vi "20TILMMonitor.vi"   [LabVIEW 2016]
uses:
  Instrument_Setup.vi
  Global/Global Variables/Data_Display_global.vi
  Equipment/Mercury iXX/Public/Libraries/Level Meter/Open/Open Level Meter Device.vi
  Equipment/Mercury iXX/Public/Libraries/Level Meter/Signals/Read/Probe Level Helium (Read).vi
  Equipment/Mercury iXX/Public/Libraries/Temperature/Open/Open Temperature Device.vi
  Equipment/Mercury iXX/Public/Libraries/Temperature/Signals/Read/Temperature (Read).vi
  Equipment/Mercury iXX/Public/Libraries/Auxiliary/Open/Open Auxiliary Device.vi
  Equipment/Mercury iXX/Public/Libraries/Auxiliary/Signals/Read/Percent Open (Read).vi
  Equipment/Mercury iXX/Public/Libraries/Pressure/Open/Open Pressure Device.vi
  Equipment/Mercury iXX/Public/Libraries/Pressure/Signals/Read/Pressure (Read).vi
  Equipment/Mercury iXX/Mercury iXX.lvlib
  Equipment/Mercury iXX/Public/Libraries/Pressure.lvlib
  Equipment/Mercury iXX/Public/Libraries/Auxiliary.lvlib
  Equipment/Mercury iXX/Public/Libraries/Temperature.lvlib
  Equipment/Mercury iXX/Public/Libraries/Level Meter.lvlib
types:
  T1 = typedef "Mercury iXX.lvlib/Mercury Reference.ctl" = cluster{"Comms":refnum<visa-resource-name>, "Device ID":string[], "Comms Layer":T2, "Command":string, "Query reference":T3}
  T2 = typedef "Mercury iXX.lvlib/Comms Transport Layer.ctl" = enum16{"Ethernet TCP/IP", "USB", "ISOBus - RS-232", "GPIB"}
  T3 = typedef "Mercury iXX.lvlib/Query Dynamic Reference.ctl" = refnum<vi>
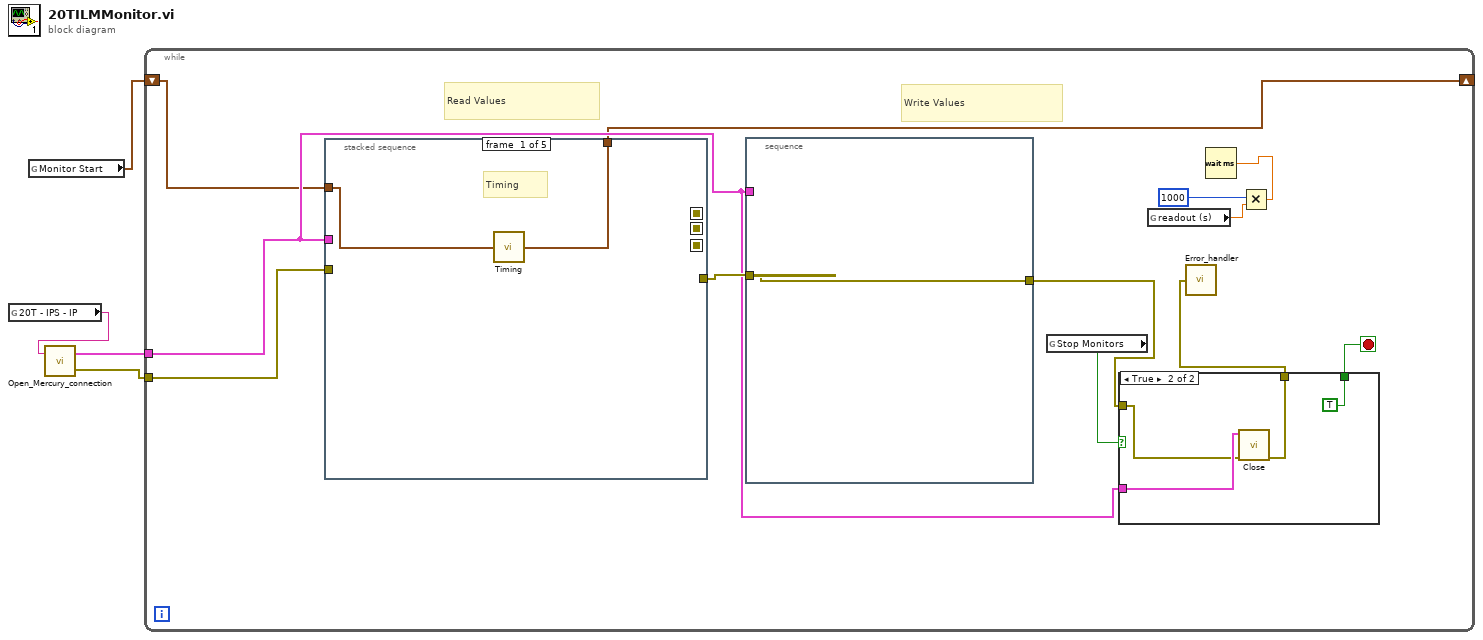
[diagram p0: block diagram]
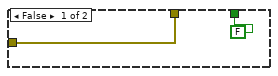
[diagram p2: hidden frame]
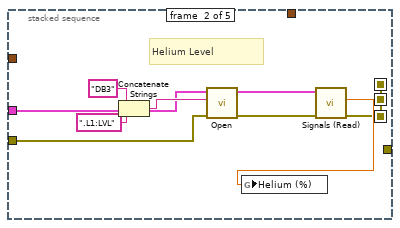
[diagram p3: hidden frame]
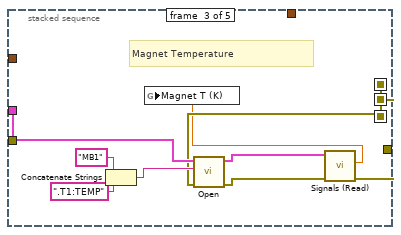
[diagram p4: hidden frame]
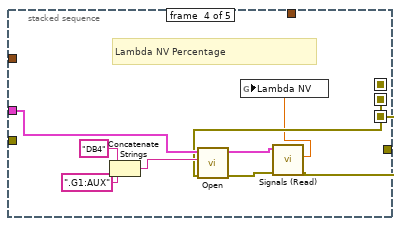
[diagram p5: hidden frame]
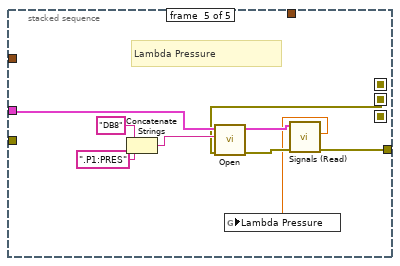
[diagram p6: hidden frame]
diagram:
  n1 = global read "Instrument_Setup.vi" "20T - IPS - IP"() -> (w2:string)
  n2 = global read "Data_Display_global.vi" "Monitor Start"() -> (w1:timestamp)
  n3 = call "Open_Mercury_connection.vi"("IP Address"=w2) -> ("error out"=w3:errorcluster, "Mercury Reference Out"=w4:T1)  [unwired: 1 in]
  n4 = while {
    tunnel: w4 -> [w7]
    tunnel: w3 -> [w16]
    shift-right: [w5] -> _
    shift-left: w1 -> [w6]
    stop <- w11 stop-if-true
    # "Write Values"
    # "Read Values"
    n5 = stacked-sequence {
      seq-local: [_ w26 _ _ _] -> [_ _ w37 _ _]
      seq-local: [_ _ w36 _ _] -> [_ _ _ w48 w57]
      seq-local: [_ _ _ w45 _] -> [_ _ _ _ _]
      tunnel: w7 -> [_ w29 w38 w49 w58]
      tunnel: w16 -> [_ w28 _ _ _]
      tunnel: [_ _ _ _ w53] -> w15
      tunnel: w6 -> [w25 _ _ _ _]
      tunnel: [w24 _ _ _ _] -> w5
      frame #0 {
        # "Timing"
        n6 = call "Timing.vi"("start time (s)"=w25) -> ("last reading (s)"=w24:timestamp)
      }
      frame #1 {
        # "Helium Level"
        n7 = Concatenate Strings("DB3", ".L1:LVL" ("Device Identifier")) -> (w32:string)
        n8 = call-poly "Open.vi"("error in (no error)"=w28, "Device Identifier"=w32, "Mercury Reference In"=w29) -> ("error out"=w34:errorcluster, "Mercury Reference Out"=w33:T1)  [unwired: 1 in, 6 out]
        n9 = call-poly "Signals (Read).vi"("error in"=w34, "Mercury Reference In"=w33) -> ("error out"=w26:errorcluster, "Level"=w27:dbl)  [unwired: 5 in, 3 out]
        n10 = global write "Data_Display_global.vi" "Helium (%)"(w27) -> ()
      }
      frame #2 {
        # "Magnet Temperature"
        n11 = Concatenate Strings("MB1", ".T1:TEMP" ("Device Identifier")) -> (w41:string)
        n12 = call-poly "Open.vi"("error in (no error)"=w37, "Device Identifier"=w41, "Mercury Reference In"=w38) -> ("error out"=w43:errorcluster, "Mercury Reference Out"=w42:T1)  [unwired: 1 in, 6 out]
        n13 = call-poly "Signals (Read).vi"("error in"=w43, "Mercury Reference In"=w42) -> ("error out"=w36:errorcluster, "Temperature"=w35:dbl)  [unwired: 5 in, 3 out]
        n14 = global write "Data_Display_global.vi" "Magnet T (K)"(w35) -> ()
      }
      frame #3 {
        # "Lambda NV Percentage"
        n15 = Concatenate Strings("DB4", ".G1:AUX" ("Device Identifier")) -> (w52:string)
        n16 = call-poly "Open.vi"("error in (no error)"=w48, "Device Identifier"=w52, "Mercury Reference In"=w49) -> ("error out"=w46:errorcluster, "Mercury Reference Out"=w47:T1)  [unwired: 1 in, 6 out]
        n17 = call-poly "Signals (Read).vi"("error in"=w46, "Mercury Reference In"=w47) -> ("error out"=w45:errorcluster, "% Open"=w44:dbl)  [unwired: 5 in, 3 out]
        n18 = global write "Data_Display_global.vi" "Lambda NV"(w44) -> ()
      }
      frame #4 {
        # "Lambda Pressure"
        n19 = Concatenate Strings("DB8", ".P1:PRES" ("Device Identifier")) -> (w61:string)
        n20 = call-poly "Open.vi"("error in (no error)"=w57, "Device Identifier"=w61, "Mercury Reference In"=w58) -> ("error out"=w55:errorcluster, "Mercury Reference Out"=w56:T1)  [unwired: 1 in, 6 out]
        n21 = call-poly "Signals (Read).vi"("error in"=w55, "Mercury Reference In"=w56) -> ("error out"=w53:errorcluster, "Temperature"=w54:dbl)  [unwired: 5 in, 3 out]
        n22 = global write "Data_Display_global.vi" "Lambda Pressure"(w54) -> ()
      }
    }
    n23 = stacked-sequence {
      tunnel: w7 -> [_]
      tunnel: w15 -> [w23]
      tunnel: [w23] -> w9
      frame #0 {
      }
    }
    n24 = global read "Data_Display_global.vi" "Stop Monitors"() -> (w10:bool)
    n25 = case shown="True" w10 {
      tunnel: w7 -> [_ w22]
      tunnel: w9 -> [w18 w21]
      tunnel: [w18 w20] -> w8
      tunnel: [FALSE TRUE] -> w11
      frame False {
      }
      frame True {
        n26 = call "Close.vi"("error in (no error)"=w21, "Mercury Reference"=w22) -> ("error out"=w20:errorcluster)  [unwired: 9 in]
      }
    }
    n27 = global read "Instrument_Setup.vi" "readout (s)"() -> (w14:dbl)
    n28 = call "Error_handler.vi"("error constant"=w8) -> ()
    n29 = Multiply(x=1000, y=w14) -> (x*y=w13:dbl)
    n30 = Wait (ms)(milliseconds to wait=w13) -> ()  [unwired: 1 out]
  }
